vi "NightM.vi"() -> ()   [LabVIEW 2010]
panel:
  in  "Path":path
  in  "Step 1":dbl
  out "error out":errorcluster
  in  "error in (no error)":errorcluster
  in  "Step 3":dbl
  in  "End 3":dbl
  in  "Start 3":dbl
  in  "Step 2":dbl
  in  "End 2":dbl
  in  "Start 2":dbl
  in  "End 1":dbl
  in  "Start 1":dbl
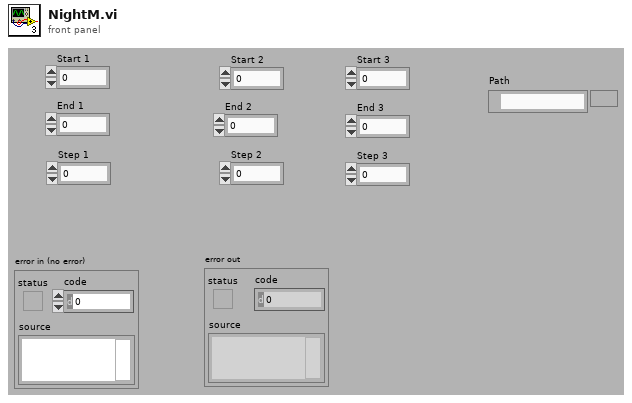
[diagram p1: front panel]
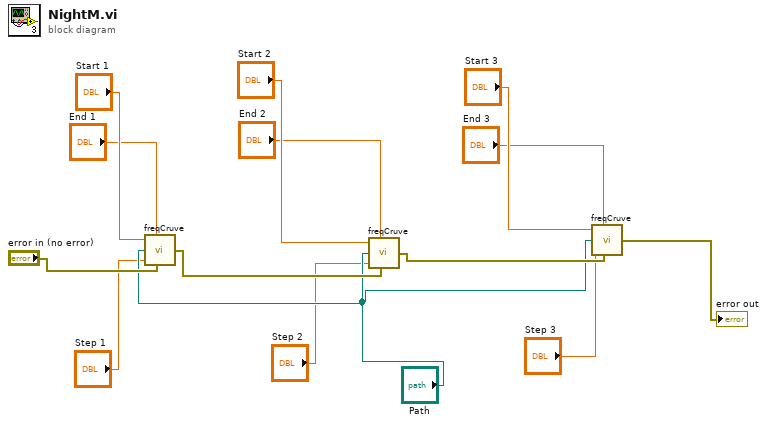
[diagram p0: block diagram]
diagram:
  n1 = call "freqCruve.vi"("Start"="Start 1", "End"="End 1", "Path"="Path", "Step"="Step 1", "error in (no error)"="error in (no error)") -> ("error out"=w13:errorcluster)
  n2 = call "freqCruve.vi"("Start"="Start 2", "End"="End 2", "Path"="Path", "Step"="Step 2", "error in (no error)"=w13) -> ("error out"=w12:errorcluster)
  n3 = call "freqCruve.vi"("Start"="Start 3", "End"="End 3", "Path"="Path", "Step"="Step 3", "error in (no error)"=w12) -> ("error out"=→"error out":errorcluster)
